vi "PingCore.vi"(8 "error in (no error)":errorcluster, 10 "Timeout (ms)":i32=-1, 11 "MicronClient in":refnum<class "MicronClient.lvclass">) -> (0 "error out":errorcluster, 2 "Response":string, 3 "MicronClient out":refnum<class "MicronClient.lvclass">)   [LabVIEW 2019, in "MicronClient.lvclass"]
uses:
  MicronClient.lvclass
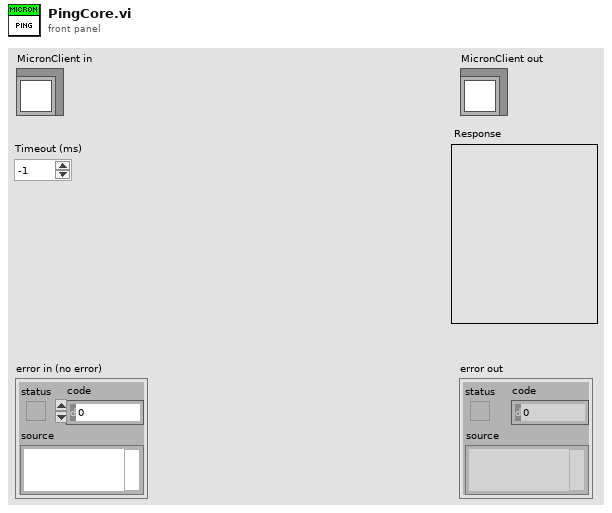
[diagram p1: front panel]
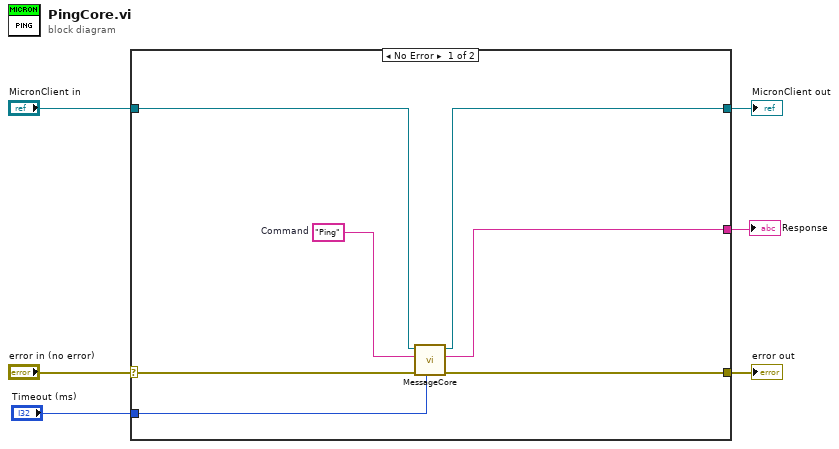
[diagram p0: block diagram]
diagram:
  n1 = case shown="No Error" "error in (no error)" {
    selector: "error in (no error)" -> [w13 w15]
    tunnel: [w12 w15] -> w5
    tunnel: [w10 w14] -> w3
    tunnel: "MicronClient in" -> [w11 w14]
    tunnel: [w8 _] -> w2
    tunnel: "Timeout (ms)" -> [w7 _]
    frame No Error {
      w9 = "Ping"  # Command
      n2 = call-dynamic "MessageCore.vi"("Timeout (ms)"=w7, "error in (no error)"=w13, "Command"=w9, "MicronClient in"=w11) -> ("error out"=w12:errorcluster, "Response"=w8:string, "MicronClient out"=w10:refnum<class "MicronClient.lvclass">)  [unwired: 5 in]
    }
    frame Error {
    }
  }
  "error out" <- w5
  "MicronClient out" <- w3
  "Response" <- w2
